vi "Binding Machine.vi"() -> ()   [LabVIEW 2014]
uses:
  Master/Master.lvclass
  Programming Logic/Programing Logic.lvclass
panel:
  out "Admin Enable":bool
  out "Drives Connection":cluster{"Drive 1":bool, "Drive 2":bool}
  in  "Delete All Record":bool
  in  "Select Record":u16(ring) items=["1", "2"]
  in  "Delete Record":bool
  out "NO.     User                   Date                 min   hr       Yields":T1(array[cluster])
  in  "Reconnect":bool
  in  "Tab Control 3":enum32{"Production", "Recipe", "Settings"}(tab)
  in  "Clear":bool
  in  "decrease":bool
  in  "Increase":bool
  out "User Yields":dbl
  in  "Zero Total Yields":bool
  out "Total Yields":dbl
  in  "Download":bool
  in  "Select Recipe":u16(ring) items=["1234567hjed", "tswri", "ad975t", "6yt"]
  in  "User 2":bool
  in  "User 1":bool
  in  "Start":bool
  in  "Stop":bool
  in  "Homing":bool
  in  "Jogging":bool
  out "Current Recipe":T2
  in  "Delete Selected Recipe":bool
  in  "Delete All Recipe":bool
  in  "Delete Recipe":u16(ring) items=["1234567hjed", "tswri", "ad975t", "6yt"]
  in  "Add Recipe":bool
  out "Index Name               Wind Leng.     Wind Spd.         Kink Cyc.        Bind Leng.        Unit":T3(array[cluster])
  in  "Set Production Page 2":bool
  in  "Set Jogging Speed":string
  in  "Display Recipe":bool
  in  "Set Auto Log off":bool
  in  "Auto Log off Time (min)":dbl
  in  "Set Admin Password":bool
  in  "Set Admin Password":T4
  out "Status":T5
  in  "Test":bool
  in  "Set Production Page":bool
  out "Time 3":dbl
  in  "Exit":bool
  out "error out":errorcluster
  in  "error in":errorcluster
  out "tab3":bool
  out "tab2":bool
  out "tab1":bool
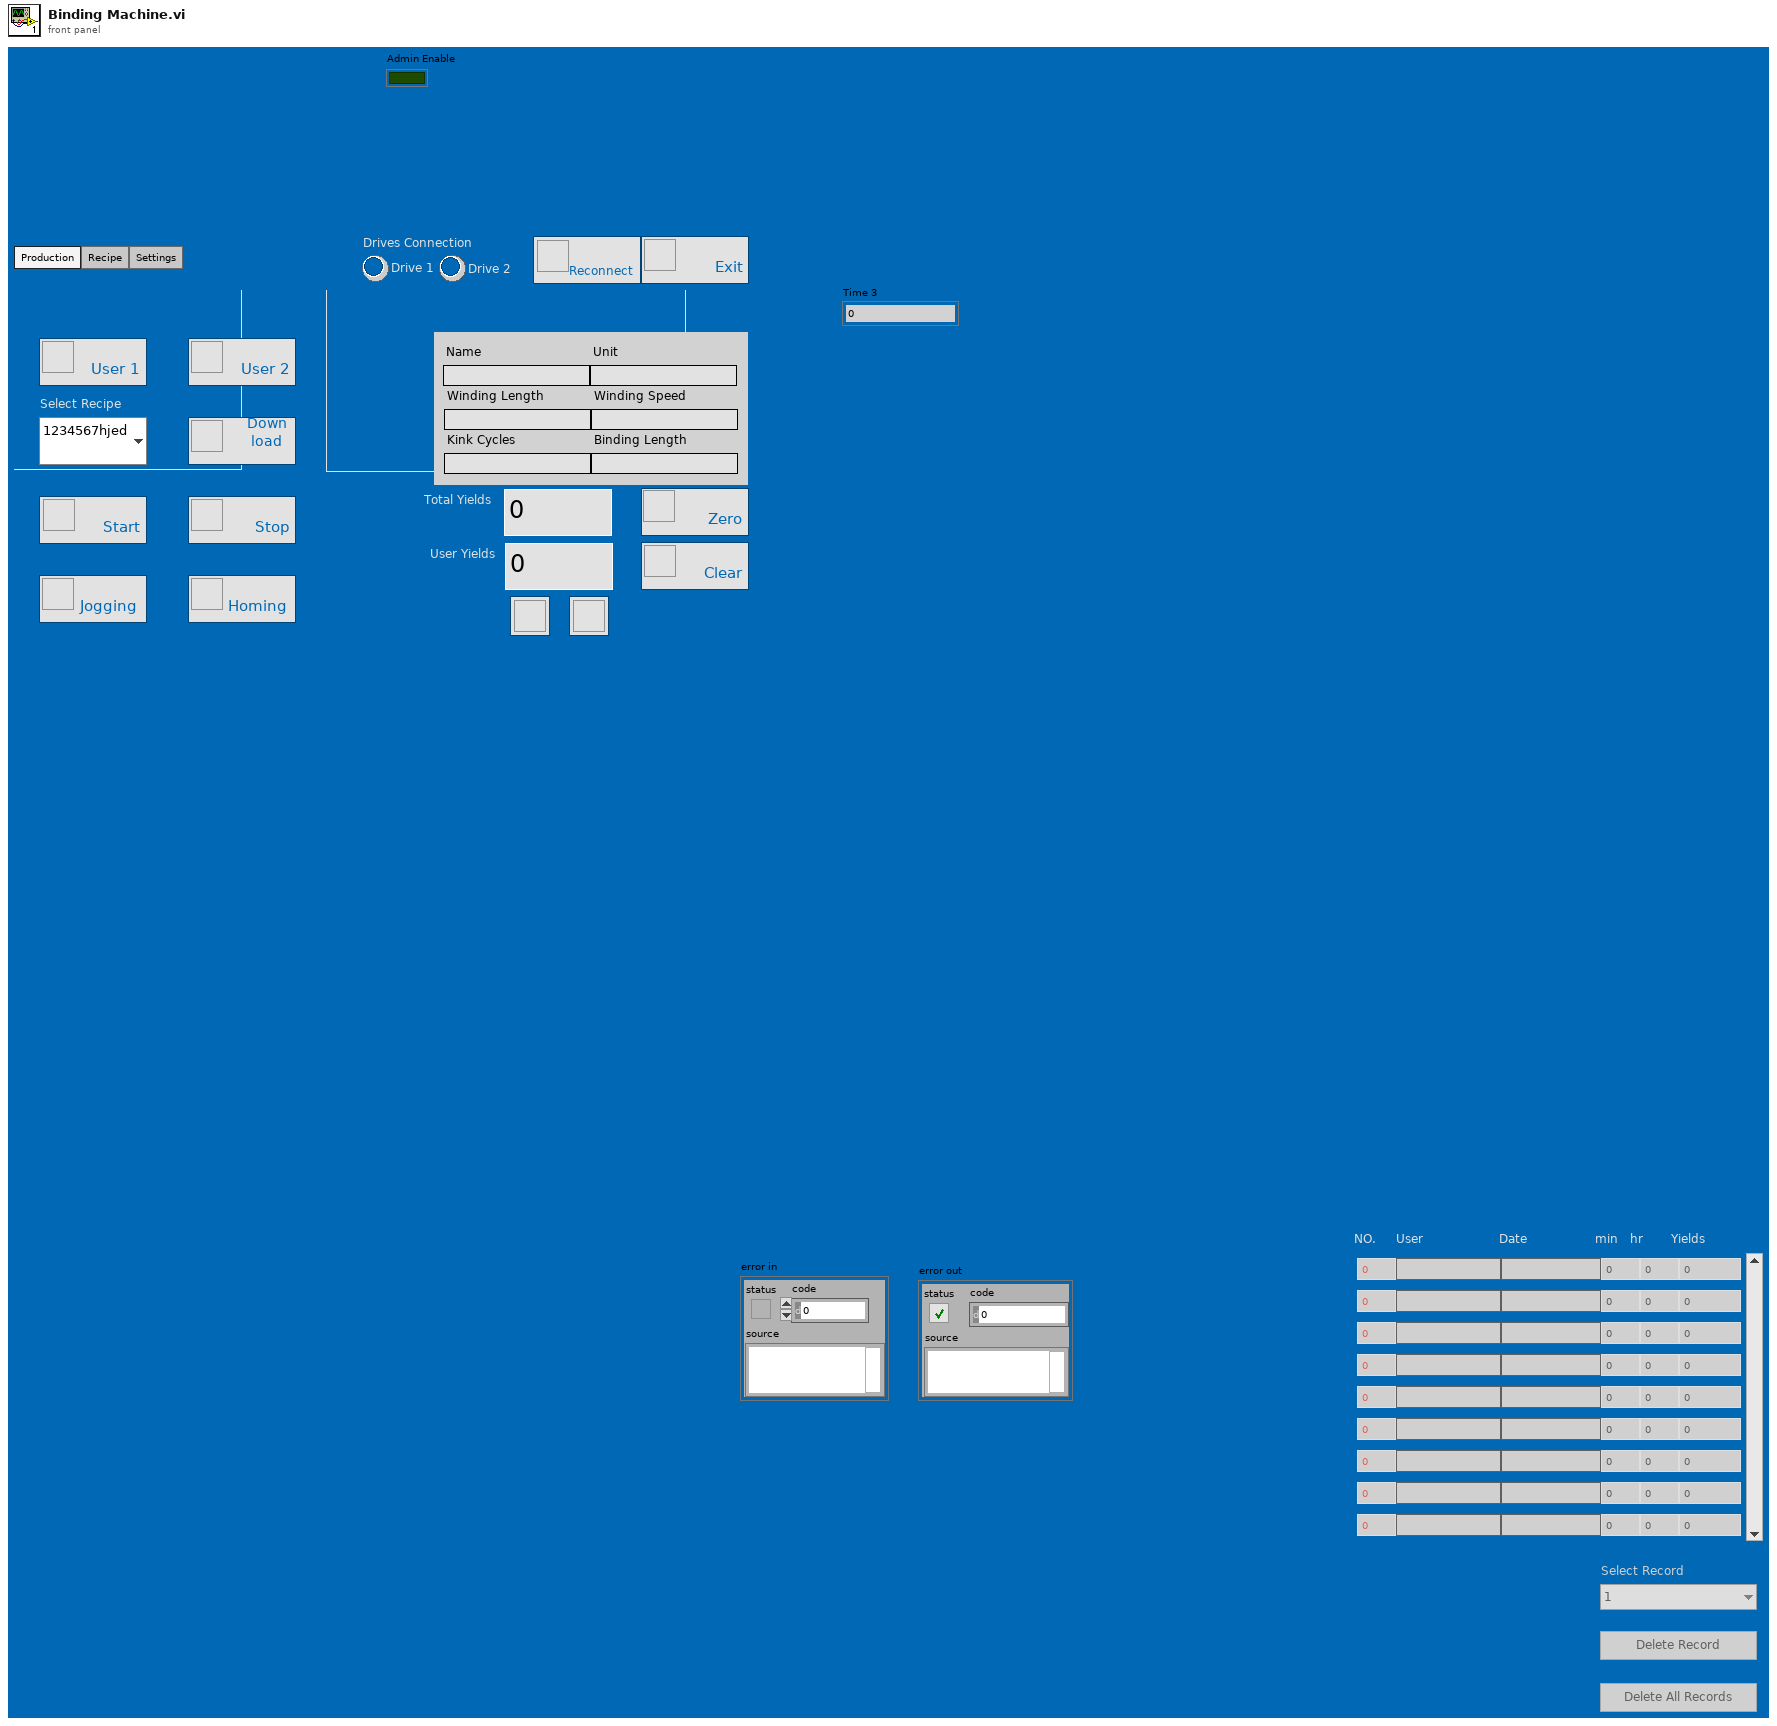
[diagram p1: front panel]
types:
  T1 = cluster{"index":i32, "User 2":string, "Date":string, "hour":i32, "min":i32, "Yields":dbl}[]
  T2 = cluster{"Name":string, "Winding Length":string, "Winding Speed":string, "Kink Cycles ":string, "Binding Length":string, "Unit":string}
  T3 = cluster{"NO.":dbl, "Name":string, "Winding Length":string, "Winding Speed":string, "Kink Cycles":string, "Binding Length":string, "Unit":string}[]
  T4 = cluster{"Old Admin Password":string, "New Admin Password":string, "Confirm  Password":string}
  T5 = cluster{"Winding":cluster{"Winding Unit":string, "Winding Speed":string, "Winding Length":string}, "Binding":cluster{"Binding Unit":string, "Kink Cycles":string, "Binding Length":string}, "Current Yields":dbl, "DataTime":cluster{"Date":string, "Time":string}, "Current User":string, "Minute":i32, "Hour":i32, "Drives Connection":cluster{"Drive 1":bool, "Drive 2":bool}}
  T6 = cluster{"Winding":cluster{"Winding Unit":string, "Winding Speed":string, "Winding Length":string}, "Binding":cluster{"Binding Unit":string, "Kink Cycles":string, "Binding Length":string}, "Yield Counts":dbl, "DataTime":cluster{"Date":string, "Time":string}, "User":string, "hour":i32, "minute":i32, "Drives Connection":cluster{"Drive 1":bool, "Drive 2":bool}}
  T7 = cluster{"Name":string, "Wind Length":string, "Wind Spd":string, "Kink Cyc":string, "Bind Length":string, "Unit":string}
  T8 = enum16{"record", "winding", "binding", "user", "recipe"}[]
  T9 = cluster{"Index":i32, "Name":string, "Wind Length":string, "Wind Spd":string, "Kink Cyc":string, "Bind Leng":string, "Unit":string}[]
  T10 = cluster{"index":i32, "User":string, "Date":string, "hour":i32, "minute":i32, "Yields":dbl}[]
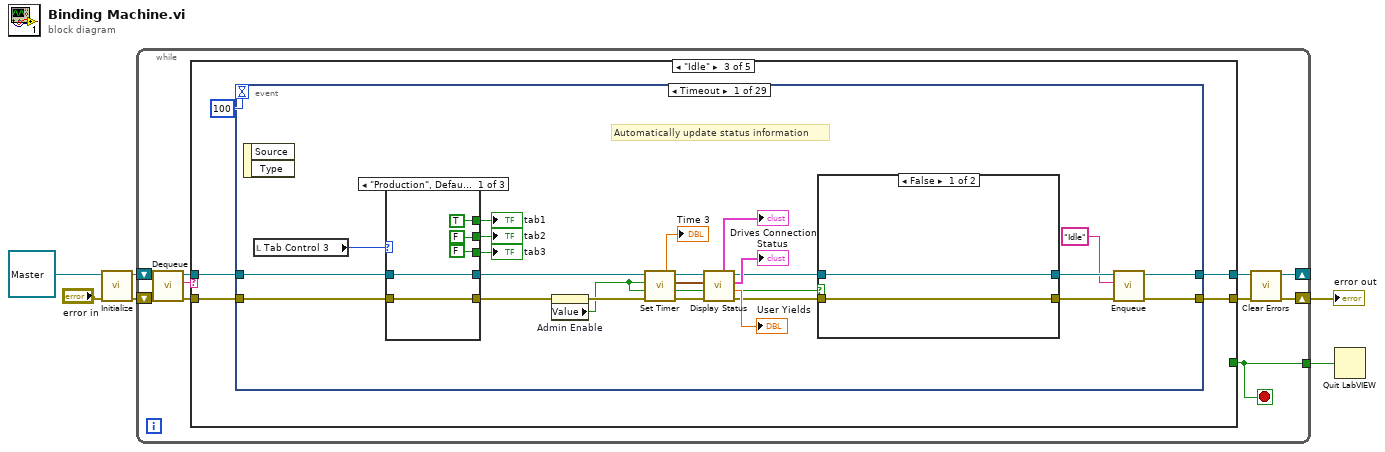
[diagram p0: block diagram]
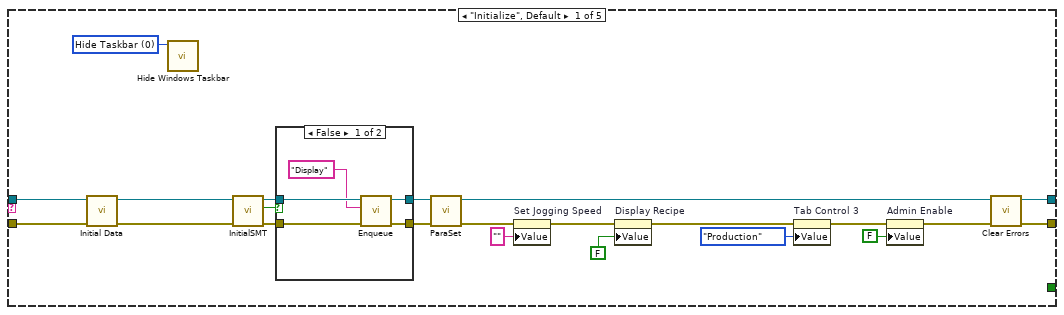
[diagram p2: hidden frame]
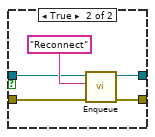
[diagram p3: hidden frame]
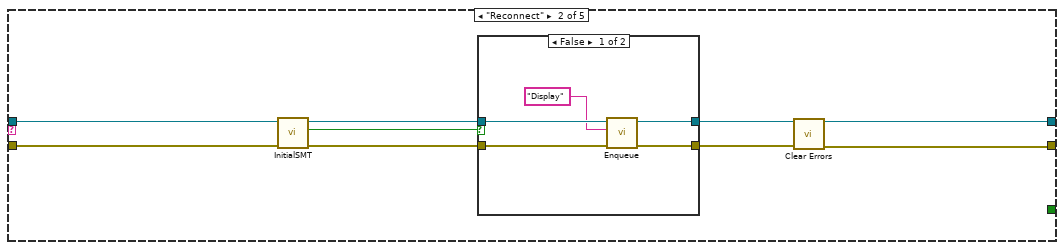
[diagram p4: hidden frame]
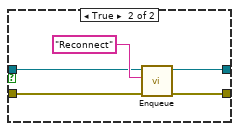
[diagram p5: hidden frame]
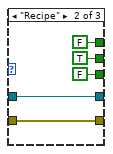
[diagram p6: hidden frame]
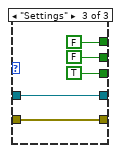
[diagram p7: hidden frame]
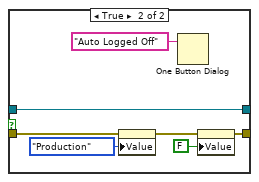
[diagram p8: hidden frame]
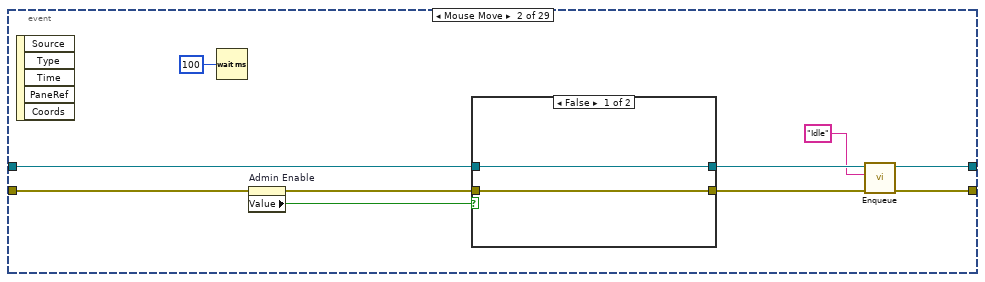
[diagram p9: hidden frame]
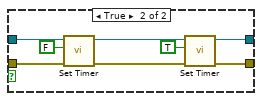
[diagram p10: hidden frame]
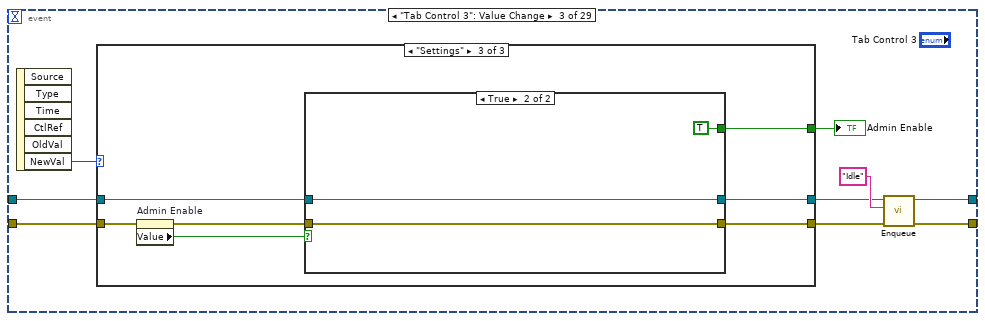
[diagram p11: hidden frame]
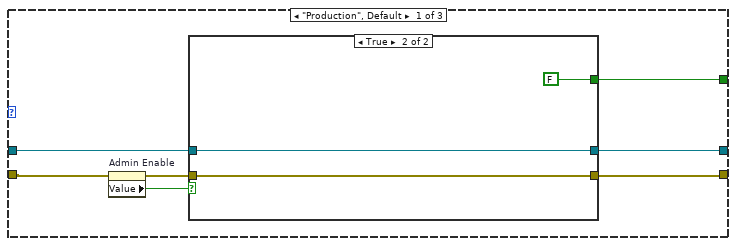
[diagram p12: hidden frame]
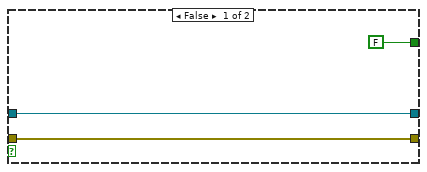
[diagram p13: hidden frame]
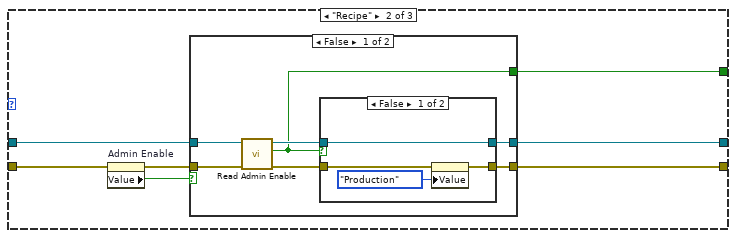
[diagram p14: hidden frame]
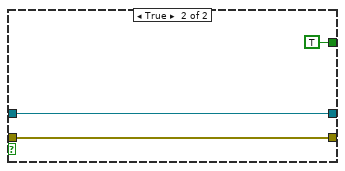
[diagram p16: hidden frame]
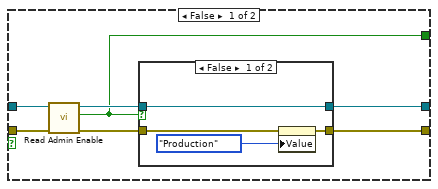
[diagram p17: hidden frame]
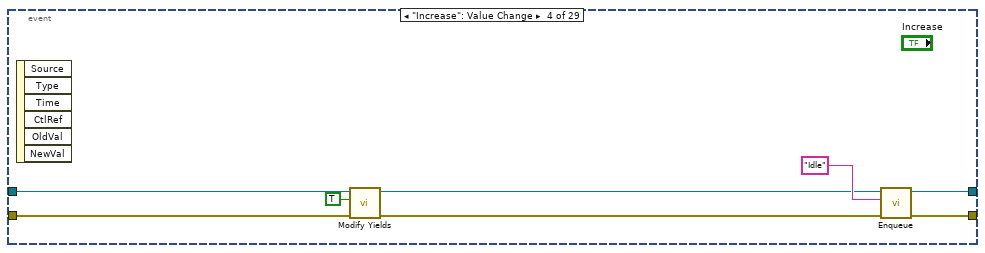
[diagram p19: hidden frame]
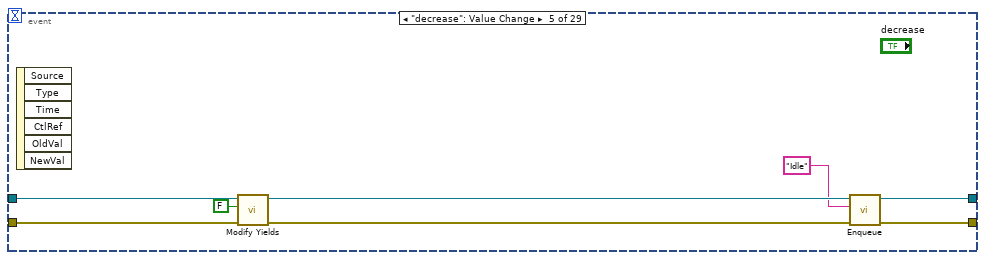
[diagram p20: hidden frame]
diagram:
  n1 = call-dynamic "Initialize.vi"("error in (no error)"="error in", "Master in"=refnum<class "Master.lvclass"> refnum ("Master.lvclass")) -> ("error out"=w4:errorcluster, "Master out"=w5:refnum<class "Master.lvclass">)  [unwired: 8 in]
  n2 = while {
    shift-right: [w11] -> _
    shift-left: w5 -> [w15]
    shift-right: [w7] -> w6
    shift-left: w4 -> [w14]
    tunnel: [w9] -> w1
    stop <- w9 stop-if-true
    n3 = call-dynamic "Dequeue.vi"("error in (no error)"=w14, "Master in"=w15) -> ("error out"=w10:errorcluster, "State"=w13:string, "Master out"=w12:refnum<class "Master.lvclass">)  [unwired: 7 in]
    n4 = case shown="\"Idle\"" w13 {
      tunnel: w12 -> [w36 w52 w69 w537 w568]
      tunnel: [w26 w50 w66 w532 w566] -> w11
      tunnel: w10 -> [w35 w51 w68 w536 w567]
      tunnel: [w16 w47 w67 w531 w565] -> w8
      tunnel: [_ _ _ _ TRUE] -> w9
      frame "Initialize", Default {
        w27 = u16 0 items=["Hide Taskbar", "Unhide Taskbar"] ("Operation")
        n5 = call-dynamic "Initial Data.vi"("error in (no error)"=w35, "Master in"=w36) -> ("error out"=w33:errorcluster, "Master out"=w34:refnum<class "Master.lvclass">)  [unwired: 8 in]
        n6 = call "Hide Windows Taskbar.vi"("Operation"=w27) -> ()  [unwired: 6 in, 1 out]
        n7 = call-dynamic "InitialSMT.vi"("error in (no error)"=w33, "Programing Logic in"=w34) -> ("error out"=w31:errorcluster, "Reconnect"=w30:bool, "Programing Logic out"=w32:refnum<class "Master.lvclass">)  [unwired: 7 in]
        n8 = case shown="False" w30 {
          tunnel: [w41 w45] -> w29
          tunnel: [w40 w44] -> w28
          tunnel: w32 -> [w39 w43]
          tunnel: w31 -> [w38 w42]
          frame False {
            n9 = call-dynamic "Enqueue.vi"("error in (no error)"=w38, "State"="Display", "Master in"=w39) -> ("error out"=w40:errorcluster, "Master out"=w41:refnum<class "Master.lvclass">)  [unwired: 7 in]
          }
          frame True {
            n10 = call-dynamic "Enqueue.vi"("error in (no error)"=w42, "State"="Reconnect", "Master in"=w43) -> ("error out"=w44:errorcluster, "Master out"=w45:refnum<class "Master.lvclass">)  [unwired: 7 in]
          }
        }
        n11 = call-dynamic "ParaSet.vi"("error in (no error)"=w28, "Programing Logic in"=w29) -> ("error out"=w22:errorcluster, "Programing Logic out"=w26:refnum<class "Master.lvclass">)  [unwired: 8 in]
        n12 = property on="Set Jogging Speed" class="Str"(error in=w22, "Value"="" ("Set Jogging Speed")) -> (error out=w21:errorcluster)  [unwired: 1 in, 1 out]
        n13 = property on="Display Recipe" class="Bool (strict)"(error in=w21, "Value"=FALSE ("Display Recipe")) -> (error out=w20:errorcluster)  [unwired: 1 in, 1 out]
        n14 = property on="Tab Control 3" class="TabCtl (strict)"(error in=w20, "Value"=enum32{"Production", "Recipe", "Settings"}."Production" ("Tab Control 3")) -> (error out=w24:errorcluster)  [unwired: 1 in, 1 out]
        n15 = property on="Admin Enable" class="Bool (strict)"(error in=w24, "Value"=FALSE ("Admin Enable")) -> (error out=w17:errorcluster)  [unwired: 1 in, 1 out]
        n16 = call <vilib>:"Clear Errors.vi"("error in (no error)"=w17) -> ("error out"=w16:errorcluster)  [unwired: 5 in, 1 out]
      }
      frame "Reconnect" {
        n17 = call-dynamic "InitialSMT.vi"("error in (no error)"=w51, "Programing Logic in"=w52) -> ("error out"=w53:errorcluster, "Reconnect"=w49:bool, "Programing Logic out"=w54:refnum<class "Master.lvclass">)  [unwired: 7 in]
        n18 = case shown="False" w49 {
          tunnel: w54 -> [w57 w63]
          tunnel: w53 -> [w56 w62]
          tunnel: [w59 w61] -> w50
          tunnel: [w58 w60] -> w48
          frame False {
            n19 = call-dynamic "Enqueue.vi"("error in (no error)"=w56, "State"="Display", "Master in"=w57) -> ("error out"=w58:errorcluster, "Master out"=w59:refnum<class "Master.lvclass">)  [unwired: 7 in]
          }
          frame True {
            n20 = call-dynamic "Enqueue.vi"("error in (no error)"=w62, "State"="Reconnect", "Master in"=w63) -> ("error out"=w60:errorcluster, "Master out"=w61:refnum<class "Master.lvclass">)  [unwired: 7 in]
          }
        }
        n21 = call <vilib>:"Clear Errors.vi"("error in (no error)"=w48) -> ("error out"=w47:errorcluster)  [unwired: 5 in, 1 out]
      }
      frame "Idle" {
        n22 = event shown="[0] Timeout" {
          selector: _ -> [_ _ _ _ _ _ _ _ _ _ _ _ _ _ _ _ _ _ _ _ _ _ _ _ _ _ _ _ _]
          dyn-events: _ -> [_ _ _ _ _ _ _ _ _ _ _ _ _ _ _ _ _ _ _ _ _ _ _ _ _ _ _ _ _]
          timeout: 100 -> [_ _ _ _ _ _ _ _ _ _ _ _ _ _ _ _ _ _ _ _ _ _ _ _ _ _ _ _ _]
          tunnel: w69 -> [w77 w127 w143 w214 w222 w224 w251 w262 w270 w284 w290 w298 w305 w312 w320 w322 w329 w344 w357 w377 w390 w407 w419 w435 w462 w498 w501 w509 w517]
          tunnel: w68 -> [w74 w124 w141 w213 w221 w223 w250 w261 w269 w275 w289 w294 w301 w308 w319 w321 w333 w343 w350 w370 w389 w406 w418 w434 w461 w497 w500 w507 w516]
          tunnel: [w82 w120 w146 w207 w217 w229 w252 w264 w272 w279 w285 w296 w303 w310 w316 w323 w331 w346 w354 w374 w391 w412 w427 w428 w467 w488 w504 w512 w521] -> w67
          tunnel: [w83 w121 w147 w208 w218 w230 w253 w265 w273 w280 w286 w297 w304 w311 w317 w324 w330 w347 w355 w375 w392 w411 w426 w429 w466 w489 w503 w511 w522] -> w66
          event Timeout {
            # "Automatically update status information"
            n23 = event-data() -> ()  [unwired: 1 in, 2 out]
            n24 = local read "Tab Control 3"() -> (w76:enum32{"Production", "Recipe", "Settings"})
            n25 = case shown="\"Production\", Default" w76 {
              tunnel: w77 -> [w99 w104 w109]
              tunnel: [w99 w104 w109] -> w75
              tunnel: [w98 w103 w108] -> w73
              tunnel: w74 -> [w98 w103 w108]
              tunnel: [TRUE FALSE FALSE] -> w72
              tunnel: [FALSE FALSE TRUE] -> w71
              tunnel: [FALSE TRUE FALSE] -> w70
              frame "Production", Default {
              }
              frame "Recipe" {
              }
              frame "Settings" {
              }
            }
            "tab1" <- w72
            "tab2" <- w70
            "tab3" <- w71
            n26 = property on="Admin Enable" class="Bool (strict)"(error in=w73) -> (error out=w86:errorcluster, "Value"=w85:bool)  [unwired: 1 in, 1 out]
            n27 = call-dynamic "Set Timer.vi"("error in (no error)"=w86, "User"=w85, "Admin"=w85, "Master in"=w75) -> ("error out"=w93:errorcluster, "Done"=w84:bool, "Cluster"=w92:cluster{"minute":i32, "hour":i32}, "Master out"=w94:refnum<class "Master.lvclass">, "Time"=→"Time 3":dbl)  [unwired: 2 in, 1 out]
            n28 = call-dynamic "Display Status.vi"("error in (no error)"=w93, "Status.Login Time"=w92, "Programing Logic in"=w94) -> ("error out"=w87:errorcluster, "commandValue"=→"User Yields":dbl, "Status"=→"Status":T6, "Programing Logic out"=w89:refnum<class "Master.lvclass">, "Drives Connection"=→"Drives Connection":cluster{"Drive 1":bool, "Drive 2":bool})  [unwired: 4 in]
            n29 = case shown="False" w84 {
              tunnel: [w110 w114] -> w80
              tunnel: [w111 w117] -> w81
              tunnel: w89 -> [w111 w117]
              tunnel: w87 -> [w110 w116]
              frame False {
              }
              frame True {
                n30 = property on="Tab Control 3" class="TabCtl (strict)"(error in=w116, "Value"=enum32{"Production", "Recipe", "Settings"}."Production" ("Tab Control 3")) -> (error out=w113:errorcluster)  [unwired: 1 in, 1 out]
                n31 = One Button Dialog(message="Auto Logged Off") -> ()  [unwired: 1 in, 1 out]
                n32 = property on="Admin Enable" class="Bool (strict)"(error in=w113, "Value"=FALSE ("Admin Enable")) -> (error out=w114:errorcluster)  [unwired: 1 in, 1 out]
              }
            }
            n33 = call-dynamic "Enqueue.vi"("error in (no error)"=w80, "State"="Idle", "Master in"=w81) -> ("error out"=w82:errorcluster, "Master out"=w83:refnum<class "Master.lvclass">)  [unwired: 7 in]
          }
          event Mouse Move {
            n34 = event-data() -> ()  [unwired: 1 in, 5 out]
            n35 = Wait (ms)(milliseconds to wait=u32 100) -> ()  [unwired: 1 out]
            n36 = property on="Admin Enable" class="Bool (strict)"(error in=w124) -> (error out=w123:errorcluster, "Value"=w125:bool)  [unwired: 1 in, 1 out]
            n37 = case shown="False" w125 {
              tunnel: w127 -> [w130 w138]
              tunnel: [w130 w136] -> w126
              tunnel: w123 -> [w129 w135]
              tunnel: [w129 w133] -> w122
              frame False {
              }
              frame True {
                n38 = call-dynamic "Set Timer.vi"("error in (no error)"=w135, "Admin"=FALSE, "Master in"=w138) -> ("error out"=w134:errorcluster, "Master out"=w137:refnum<class "Master.lvclass">)  [unwired: 3 in, 4 out]
                n39 = call-dynamic "Set Timer.vi"("error in (no error)"=w134, "Admin"=TRUE, "Master in"=w137) -> ("error out"=w133:errorcluster, "Master out"=w136:refnum<class "Master.lvclass">)  [unwired: 3 in, 4 out]
              }
            }
            n40 = call-dynamic "Enqueue.vi"("error in (no error)"=w122, "State"="Idle", "Master in"=w126) -> ("error out"=w120:errorcluster, "Master out"=w121:refnum<class "Master.lvclass">)  [unwired: 7 in]
          }
          event "Tab Control 3": Value Change {
            n41 = event-data() -> ("NewVal"=w144:enum32{"Production", "Recipe", "Settings"})  [unwired: 1 in, 5 out]
            n42 = case shown="\"Settings\"" w144 {
              tunnel: w143 -> [w152 w167 w189]
              tunnel: [w151 w166 w190] -> w142
              tunnel: w141 -> [w154 w164 w187]
              tunnel: [w149 w165 w185] -> w140
              tunnel: [w148 w161 w184] -> w139
              frame "Production", Default {
                n43 = property on="Admin Enable" class="Bool (strict)"(error in=w154) -> (error out=w150:errorcluster, "Value"=w153:bool)  [unwired: 1 in, 1 out]
                n44 = case shown="True" w153 {
                  tunnel: w152 -> [w157 w160]
                  tunnel: [w157 w160] -> w151
                  tunnel: [w156 w158] -> w149
                  tunnel: w150 -> [w156 w158]
                  tunnel: [FALSE ("Admin Enable") FALSE ("Admin Enable")] -> w148
                  frame False {
                  }
                  frame True {
                  }
                }
              }
              frame "Recipe" {
                n45 = property on="Admin Enable" class="Bool (strict)"(error in=w164) -> (error out=w163:errorcluster, "Value"=w162:bool)  [unwired: 1 in, 1 out]
                n46 = case shown="False" w162 {
                  tunnel: w167 -> [w174 w183]
                  tunnel: [w171 w183] -> w166
                  tunnel: [w169 w182] -> w165
                  tunnel: w163 -> [w173 w182]
                  tunnel: [w168 TRUE ("Admin Enable")] -> w161
                  frame False {
                    n47 = call-dynamic "Read Admin Enable.vi"("error in (no error)"=w173, "Master in"=w174) -> ("error out"=w170:errorcluster, "Admin Enable"=w168:bool, "Master out"=w172:refnum<class "Master.lvclass">)  [unwired: 4 in, 3 out]
                    n48 = case shown="False" w168 {
                      tunnel: [w178 w180] -> w171
                      tunnel: w172 -> [w178 w180]
                      tunnel: [w177 w179] -> w169
                      tunnel: w170 -> [w176 w179]
                      frame False {
                        n49 = property on="Tab Control 3" class="TabCtl (strict)"(error in=w176, "Value"=enum32{"Production", "Recipe", "Settings"}."Production" ("Tab Control 3")) -> (error out=w177:errorcluster)  [unwired: 1 in, 1 out]
                      }
                      frame True {
                      }
                    }
                  }
                  frame True {
                  }
                }
              }
              frame "Settings" {
                n50 = property on="Admin Enable" class="Bool (strict)"(error in=w187) -> (error out=w188:errorcluster, "Value"=w186:bool)  [unwired: 1 in, 1 out]
                n51 = case shown="True" w186 {
                  tunnel: w189 -> [w197 w206]
                  tunnel: [w194 w206] -> w190
                  tunnel: [w192 w205] -> w185
                  tunnel: w188 -> [w196 w205]
                  tunnel: [w191 TRUE ("Admin Enable")] -> w184
                  frame False {
                    n52 = call-dynamic "Read Admin Enable.vi"("error in (no error)"=w196, "Master in"=w197) -> ("error out"=w193:errorcluster, "Admin Enable"=w191:bool, "Master out"=w195:refnum<class "Master.lvclass">)  [unwired: 4 in, 3 out]
                    n53 = case shown="False" w191 {
                      tunnel: [w201 w203] -> w194
                      tunnel: w195 -> [w201 w203]
                      tunnel: [w200 w202] -> w192
                      tunnel: w193 -> [w199 w202]
                      frame False {
                        n54 = property on="Tab Control 3" class="TabCtl (strict)"(error in=w199, "Value"=enum32{"Production", "Recipe", "Settings"}."Production" ("Tab Control 3")) -> (error out=w200:errorcluster)  [unwired: 1 in, 1 out]
                      }
                      frame True {
                      }
                    }
                  }
                  frame True {
                  }
                }
              }
            }
            "Admin Enable" <- w139
            n55 = call-dynamic "Enqueue.vi"("error in (no error)"=w140, "State"="Idle", "Master in"=w142) -> ("error out"=w146:errorcluster, "Master out"=w147:refnum<class "Master.lvclass">)  [unwired: 7 in]
          }
          event "Increase": Value Change {
            n56 = event-data() -> ()  [unwired: 1 in, 6 out]
            n57 = call-dynamic "Modify Yields.vi"("error in (no error)"=w213, "Boolean"=TRUE, "Programing Logic in"=w214) -> ("error out"=w209:errorcluster, "Programing Logic out"=w210:refnum<class "Master.lvclass">)  [unwired: 7 in]
            n58 = call-dynamic "Enqueue.vi"("error in (no error)"=w209, "State"="Idle", "Master in"=w210) -> ("error out"=w207:errorcluster, "Master out"=w208:refnum<class "Master.lvclass">)  [unwired: 7 in]
          }
          event "decrease": Value Change {
            n59 = event-data() -> ()  [unwired: 1 in, 6 out]
            n60 = call-dynamic "Modify Yields.vi"("error in (no error)"=w221, "Boolean"=FALSE, "Programing Logic in"=w222) -> ("error out"=w219:errorcluster, "Programing Logic out"=w220:refnum<class "Master.lvclass">)  [unwired: 7 in]
            n61 = call-dynamic "Enqueue.vi"("error in (no error)"=w219, "State"="Idle", "Master in"=w220) -> ("error out"=w217:errorcluster, "Master out"=w218:refnum<class "Master.lvclass">)  [unwired: 7 in]
          }
          event "Zero Total Yields": Value Change {
            n62 = event-data() -> ()  [unwired: 1 in, 6 out]
            n63 = Two Button Dialog(message="Zero Total Yields?", 1:"No" ("F button name (\"Cancel\")"), 2:"Yes" ("T button name (\"OK\")")) -> (T button?=w228:bool)
            n64 = case shown="True" w228 {
              tunnel: [w234 w246] -> w230
              tunnel: [w233 w245] -> w229
              tunnel: w224 -> [w232 w237]
              tunnel: w223 -> [w231 w236]
              frame False {
                n65 = call-dynamic "Enqueue.vi"("error in (no error)"=w231, "State"="Idle", "Master in"=w232) -> ("error out"=w233:errorcluster, "Master out"=w234:refnum<class "Master.lvclass">)  [unwired: 7 in]
              }
              frame True {
                n66 = call-dynamic "Path.vi"("error in (no error)"=w236, "pathname"="production record", "Master in"=w237) -> ("error out"=w242:errorcluster, "Master out"=w243:refnum<class "Master.lvclass">)  [unwired: 7 in]
                n67 = call-dynamic "Zero Yields.vi"("error in (no error)"=w242, "Master in"=w243) -> ("error out"=w240:errorcluster, "Master out"=w241:refnum<class "Master.lvclass">)  [unwired: 8 in]
                n68 = call-dynamic "WriteFiles.vi"("error in (no error)"=w240, "Master in"=w241) -> ("error out"=w238:errorcluster, "Master out"=w239:refnum<class "Master.lvclass">)  [unwired: 8 in]
                n69 = call-dynamic "Enqueue.vi"("error in (no error)"=w238, "State"="Display", "Master in"=w239) -> ("error out"=w245:errorcluster, "Master out"=w246:refnum<class "Master.lvclass">)  [unwired: 7 in]
              }
            }
          }
          event "Clear": Value Change {
            n70 = event-data() -> ()  [unwired: 1 in, 6 out]
            n71 = call-dynamic "Zero.vi"("error in (no error)"=w250, "Programing Logic in"=w251) -> ("error out"=w248:errorcluster, "Programing Logic out"=w249:refnum<class "Master.lvclass">)  [unwired: 8 in]
            n72 = call-dynamic "Enqueue.vi"("error in (no error)"=w248, "Master in"=w249) -> ("error out"=w252:errorcluster, "Master out"=w253:refnum<class "Master.lvclass">)  [unwired: 8 in]
          }
          event "Set Auto Log off": Value Change {
            # "Set auto log off time by adminstrator only"
            n73 = event-data() -> ()  [unwired: 1 in, 6 out]
            n74 = call-dynamic "Set Auto Logoff.vi"("error in (no error)"=w261, "Timer.AutoLogoff"="Auto Log off Time (min)", "Master in"=w262) -> ("error out"=w259:errorcluster, "Master out"=w260:refnum<class "Master.lvclass">)  [unwired: 7 in]
            n75 = call-dynamic "Path.vi"("error in (no error)"=w259, "pathname"="login", "Master in"=w260) -> ("error out"=w257:errorcluster, "Master out"=w258:refnum<class "Master.lvclass">)  [unwired: 7 in]
            n76 = call-dynamic "WriteFiles.vi"("error in (no error)"=w257, "Master in"=w258) -> ("error out"=w255:errorcluster, "Master out"=w256:refnum<class "Master.lvclass">)  [unwired: 8 in]
            n77 = call-dynamic "Enqueue.vi"("error in (no error)"=w255, "State"="Idle", "Master in"=w256) -> ("error out"=w264:errorcluster, "Master out"=w265:refnum<class "Master.lvclass">)  [unwired: 7 in]
          }
          event "Add Recipe": Value Change {
            n78 = event-data() -> ()  [unwired: 1 in, 1 out]
            n79 = call-dynamic "Add Recipe.vi"("error in (no error)"=w269, "Master in"=w270) -> ("error out"=w267:errorcluster, "Master out"=w268:refnum<class "Master.lvclass">)  [unwired: 8 in]
            n80 = call-dynamic "Enqueue.vi"("error in (no error)"=w267, "State"="Display", "Master in"=w268) -> ("error out"=w272:errorcluster, "Master out"=w273:refnum<class "Master.lvclass">)  [unwired: 7 in]
          }
          event "Download": Value Change {
            n81 = event-data() -> ()  [unwired: 1 in, 1 out]
            n82 = call-dynamic "Download Recipe.vi"("index"="Select Recipe", "error in (no error)"=w275, "Master in"=w284) -> ("error out"=w281:errorcluster, "Parameter"=w282:T7, "Master out"=w283:refnum<class "Master.lvclass">)  [unwired: 6 in]
            n83 = call-dynamic "Download Recipe_galil.vi"("error in (no error)"=w281, "Parameter"=w282, "Programing Logic in"=w283) -> ("error out"=w276:errorcluster, "Programing Logic out"=w277:refnum<class "Master.lvclass">)  [unwired: 7 in]
            n84 = call-dynamic "Enqueue.vi"("error in (no error)"=w276, "State"="Display", "Master in"=w277) -> ("error out"=w279:errorcluster, "Master out"=w280:refnum<class "Master.lvclass">)  [unwired: 7 in]
          }
          event "Set Production Page 2": Value Change {
            n85 = event-data() -> ()  [unwired: 1 in, 1 out]
            n86 = call-dynamic "Display Recipe Enable.vi"("error in (no error)"=w289, "Display Recipe"="Display Recipe", "Master in"=w290) -> ("error out"=w287:errorcluster, "Master out"=w288:refnum<class "Master.lvclass">)  [unwired: 7 in]
            n87 = call-dynamic "Enqueue.vi"("error in (no error)"=w287, "State"="Display", "Master in"=w288) -> ("error out"=w285:errorcluster, "Master out"=w286:refnum<class "Master.lvclass">)  [unwired: 7 in]
          }
          event "Set Admin Password.Old Admin Password": Mouse Down {
            n88 = event-data() -> ()  [unwired: 1 in, 1 out]
            n89 = call "numberpad.vi"() -> ("String"=w293:string)  [unwired: 11 in]
            n90 = property on="Old Admin Password" class="Str"(error in=w294, "Value"=w293) -> (error out=w295:errorcluster)  [unwired: 1 in, 1 out]
            n91 = call-dynamic "Enqueue.vi"("error in (no error)"=w295, "State"="Idle", "Master in"=w298) -> ("error out"=w296:errorcluster, "Master out"=w297:refnum<class "Master.lvclass">)  [unwired: 7 in]
          }
          event "Set Admin Password.New Admin Password": Mouse Down {
            n92 = event-data() -> ()  [unwired: 1 in, 1 out]
            n93 = call "numberpad.vi"() -> ("String"=w300:string)  [unwired: 11 in]
            n94 = property on="New Admin Password" class="Str"(error in=w301, "Value"=w300) -> (error out=w302:errorcluster)  [unwired: 1 in, 1 out]
            n95 = call-dynamic "Enqueue.vi"("error in (no error)"=w302, "State"="Idle", "Master in"=w305) -> ("error out"=w303:errorcluster, "Master out"=w304:refnum<class "Master.lvclass">)  [unwired: 7 in]
          }
          event "Set Admin Password.Confirm  Password": Mouse Down {
            n96 = event-data() -> ()  [unwired: 1 in, 1 out]
            n97 = call "numberpad.vi"() -> ("String"=w307:string)  [unwired: 11 in]
            n98 = property on="Confirm  Password" class="Str"(error in=w308, "Value"=w307) -> (error out=w309:errorcluster)  [unwired: 1 in, 1 out]
            n99 = call-dynamic "Enqueue.vi"("error in (no error)"=w309, "State"="Idle", "Master in"=w312) -> ("error out"=w310:errorcluster, "Master out"=w311:refnum<class "Master.lvclass">)  [unwired: 7 in]
          }
          event "Test": Value Change {
            n100 = event-data() -> ()  [unwired: 1 in, 1 out]
            n101 = call-dynamic "Motor Test.vi"("error in (no error)"=w319, "Programing Logic in"=w320) -> ("error out"=w314:errorcluster, "Programing Logic out"=w315:refnum<class "Master.lvclass">)  [unwired: 8 in]
            n102 = call-dynamic "Enqueue.vi"("error in (no error)"=w314, "State"="Idle", "Master in"=w315) -> ("error out"=w316:errorcluster, "Master out"=w317:refnum<class "Master.lvclass">)  [unwired: 7 in]
          }
          event "Set Production Page": Value Change {
            n103 = event-data() -> ()  [unwired: 1 in, 1 out]
            n104 = call-dynamic "Set Jogging Spd.vi"("error in (no error)"=w321, "Set Jogging Speed"="Set Jogging Speed", "Programing Logic in"=w322) -> ("error out"=w325:errorcluster, "Programing Logic out"=w326:refnum<class "Master.lvclass">)  [unwired: 7 in]
            n105 = call-dynamic "Enqueue.vi"("error in (no error)"=w325, "State"="Display", "Master in"=w326) -> ("error out"=w323:errorcluster, "Master out"=w324:refnum<class "Master.lvclass">)  [unwired: 7 in]
          }
          event "Set Jogging Speed": Mouse Down {
            n106 = event-data() -> ()  [unwired: 1 in, 1 out]
            n107 = call "numberpad.vi"() -> ("String"=w334:string)  [unwired: 11 in]
            n108 = property on="Set Jogging Speed" class="Str"(error in=w333, "Value"=w334) -> (error out=w332:errorcluster)  [unwired: 1 in, 1 out]
            n109 = call-dynamic "Enqueue.vi"("error in (no error)"=w332, "State"="Idle", "Master in"=w329) -> ("error out"=w331:errorcluster, "Master out"=w330:refnum<class "Master.lvclass">)  [unwired: 7 in]
          }
          event "Delete Record": Value Change {
            n110 = event-data() -> ()  [unwired: 1 in, 1 out]
            n111 = call-dynamic "Path.vi"("error in (no error)"=w343, "pathname"="production record", "Master in"=w344) -> ("error out"=w339:errorcluster, "Master out"=w340:refnum<class "Master.lvclass">)  [unwired: 7 in]
            n112 = call-dynamic "Delete Record.vi"("index"="Select Record", "error in (no error)"=w339, "Master in"=w340) -> ("error out"=w337:errorcluster, "Master out"=w338:refnum<class "Master.lvclass">)  [unwired: 7 in]
            n113 = call-dynamic "WriteFiles.vi"("error in (no error)"=w337, "Master in"=w338) -> ("error out"=w341:errorcluster, "Master out"=w342:refnum<class "Master.lvclass">)  [unwired: 8 in]
            n114 = call-dynamic "Enqueue.vi"("error in (no error)"=w341, "State"="Display", "Master in"=w342) -> ("error out"=w346:errorcluster, "Master out"=w347:refnum<class "Master.lvclass">)  [unwired: 7 in]
          }
          event "User 1": Value Change {
            n115 = event-data() -> ()  [unwired: 1 in, 2 out]
            n116 = property on="User 1" class="Bool (strict)"(error in=w350) -> (error out=w351:errorcluster, "Value"=w349:bool)  [unwired: 1 in, 1 out]
            n117 = case shown="False" w349 {
              tunnel: w357 -> [w361 w367]
              tunnel: w351 -> [w359 w366]
              tunnel: [w360 w365] -> w353
              tunnel: [w361 w362] -> w352
              frame False {
                n118 = property on="User 1" class="Bool (strict)"(error in=w359, "Value"=TRUE ("User 1")) -> (error out=w360:errorcluster)  [unwired: 1 in, 1 out]
              }
              frame True {
                n119 = call-dynamic "Load User.vi"("User Name 2"="User 1", "error in (no error)"=w366, "Programing Logic in"=w367) -> ("error out"=w364:errorcluster, "Programing Logic out"=w362:refnum<class "Master.lvclass">)  [unwired: 7 in]
                n120 = property on="User 2" class="Bool (strict)"(error in=w364, "Value"=FALSE ("User 2")) -> (error out=w365:errorcluster)  [unwired: 1 in, 1 out]
              }
            }
            n121 = call-dynamic "Enqueue.vi"("error in (no error)"=w353, "State"="Idle", "Master in"=w352) -> ("error out"=w354:errorcluster, "Master out"=w355:refnum<class "Master.lvclass">)  [unwired: 7 in]
          }
          event "User 2": Value Change {
            n122 = event-data() -> ()  [unwired: 1 in, 2 out]
            n123 = property on="User 2" class="Bool (strict)"(error in=w370) -> (error out=w371:errorcluster, "Value"=w369:bool)  [unwired: 1 in, 1 out]
            n124 = case shown="False" w369 {
              tunnel: w377 -> [w381 w388]
              tunnel: w371 -> [w379 w387]
              tunnel: [w381 w385] -> w373
              tunnel: [w380 w384] -> w372
              frame False {
                n125 = property on="User 2" class="Bool (strict)"(error in=w379, "Value"=TRUE ("User 2")) -> (error out=w380:errorcluster)  [unwired: 1 in, 1 out]
              }
              frame True {
                n126 = call-dynamic "Load User.vi"("User Name 2"="User 2", "error in (no error)"=w387, "Programing Logic in"=w388) -> ("error out"=w383:errorcluster, "Programing Logic out"=w385:refnum<class "Master.lvclass">)  [unwired: 7 in]
                n127 = property on="User 1" class="Bool (strict)"(error in=w383, "Value"=FALSE ("User 2")) -> (error out=w384:errorcluster)  [unwired: 1 in, 1 out]
              }
            }
            n128 = call-dynamic "Enqueue.vi"("error in (no error)"=w372, "State"="Idle", "Master in"=w373) -> ("error out"=w374:errorcluster, "Master out"=w375:refnum<class "Master.lvclass">)  [unwired: 7 in]
          }
          event "Reconnect": Value Change {
            n129 = event-data() -> ()  [unwired: 1 in, 2 out]
            n130 = call-dynamic "InitialSMT.vi"("error in (no error)"=w389, "Programing Logic in"=w390) -> ("error out"=w394:errorcluster, "Reconnect"=w395:bool, "Programing Logic out"=w393:refnum<class "Master.lvclass">)  [unwired: 7 in]
            n131 = case shown="True" w395 {
              tunnel: w393 -> [w398 w404]
              tunnel: w394 -> [w397 w403]
              tunnel: [w400 w402] -> w392
              tunnel: [w399 w401] -> w391
              frame False {
                n132 = call-dynamic "Enqueue.vi"("error in (no error)"=w397, "State"="Display", "Master in"=w398) -> ("error out"=w399:errorcluster, "Master out"=w400:refnum<class "Master.lvclass">)  [unwired: 7 in]
              }
              frame True {
                n133 = call-dynamic "Enqueue.vi"("error in (no error)"=w403, "State"="Reconnect", "Master in"=w404) -> ("error out"=w401:errorcluster, "Master out"=w402:refnum<class "Master.lvclass">)  [unwired: 7 in]
              }
            }
          }
          event "Exit": Value Change {
            n134 = event-data() -> ()  [unwired: 1 in, 6 out]
            n135 = call "Emergency Stop.vi"("error in (no error)"=w406, "Programing Logic in"=w407) -> ("error out"=w408:errorcluster, "Programing Logic out"=w409:refnum<class "Master.lvclass">)  [unwired: 8 in]
            n136 = call-dynamic "Enqueue.vi"("error in (no error)"=w408, "State"="Exit", "Master in"=w409) -> ("error out"=w412:errorcluster, "Master out"=w411:refnum<class "Master.lvclass">)  [unwired: 7 in]
          }
          event "Set Admin Password": Value Change {
            n137 = event-data() -> ()  [unwired: 1 in, 1 out]
            n138 = call-dynamic "Set Admin Password.vi"("error in (no error)"=w418, "Set New Admin Password"="Set Admin Password", "Master in"=w419) -> ("error out"=w417:errorcluster, "Master out"=w420:refnum<class "Master.lvclass">)  [unwired: 7 in]
            n139 = call-dynamic "Path.vi"("error in (no error)"=w417, "pathname"="login" ("Recipes"), "Master in"=w420) -> ("error out"=w421:errorcluster, "Master out"=w422:refnum<class "Master.lvclass">)  [unwired: 7 in]
            n140 = call-dynamic "WriteFiles.vi"("error in (no error)"=w421, "Master in"=w422) -> ("error out"=w415:errorcluster, "Master out"=w423:refnum<class "Master.lvclass">)  [unwired: 8 in]
            n141 = property on="Set Admin Password" class="Clust (strict)"(error in=w415, "Value"=cluster{string, string, string} {"", "", ""}) -> (error out=w414:errorcluster)  [unwired: 1 in, 1 out]
            n142 = call-dynamic "Enqueue.vi"("error in (no error)"=w414, "State"="Idle", "Master in"=w423) -> ("error out"=w427:errorcluster, "Master out"=w426:refnum<class "Master.lvclass">)  [unwired: 7 in]
          }
          event "Delete All Recipe": Value Change {
            n143 = event-data() -> ()  [unwired: 1 in, 1 out]
            n144 = Two Button Dialog(message="Delete All Recipes?", 1:"No" ("F button name (\"Cancel\")"), 2:"Yes" ("T button name (\"OK\")")) -> (T button?=w433:bool)
            n145 = case shown="True" w433 {
              tunnel: w435 -> [w440 w451]
              tunnel: w434 -> [w439 w450]
              tunnel: [w440 w444] -> w431
              tunnel: [w439 w443] -> w430
              frame False {
              }
              frame True {
                n146 = local read "Index Name               Wind Leng.     Wind Spd.         Kink Cyc.        Bind Leng.        Unit"() -> (w448:T3)
                n147 = Array Size(array=w448) -> (size(s)=w449:i32)
                n148 = for {
                  N: w449 -> [_]
                  shift-right: [w456] -> w447
                  shift-left: w451 -> [w454]
                  shift-right: [w455] -> w446
                  shift-left: w450 -> [w453]
                  n149 = call-dynamic "Delete Recipe.vi"("error in (no error)"=w453, "index"=0, "Master in"=w454) -> ("error out"=w455:errorcluster, "Master out"=w456:refnum<class "Master.lvclass">)  [unwired: 7 in]
                }
                n150 = call-dynamic "Path.vi"("error in (no error)"=w446, "pathname"="Recipes", "Master in"=w447) -> ("error out"=w441:errorcluster, "Master out"=w442:refnum<class "Master.lvclass">)  [unwired: 7 in]
                n151 = call-dynamic "WriteFiles.vi"("error in (no error)"=w441, "Master in"=w442) -> ("error out"=w443:errorcluster, "Master out"=w444:refnum<class "Master.lvclass">)  [unwired: 8 in]
              }
            }
            n152 = call-dynamic "Enqueue.vi"("error in (no error)"=w430, "State"="Display", "Master in"=w431) -> ("error out"=w428:errorcluster, "Master out"=w429:refnum<class "Master.lvclass">)  [unwired: 7 in]
          }
          event "Delete All Record": Value Change {
            n153 = event-data() -> ()  [unwired: 1 in, 1 out]
            n154 = Two Button Dialog(message="Delete All Records?", 1:"No" ("F button name (\"Cancel\")"), 2:"Yes" ("T button name (\"OK\")")) -> (T button?=w457:bool)
            n155 = case shown="True" w457 {
              tunnel: [w468 w474] -> w464
              tunnel: [w469 w479] -> w463
              tunnel: w462 -> [w468 w478]
              tunnel: w461 -> [w469 w476]
              frame False {
              }
              frame True {
                n156 = local read "NO.     User                   Date                 min   hr       Yields"() -> (w470:T1)
                n157 = Array Size(array=w470) -> (size(s)=w471:i32)
                n158 = for {
                  N: w471 -> [_]
                  shift-right: [w484] -> w477
                  shift-left: w478 -> [w485]
                  shift-right: [w482] -> w475
                  shift-left: w476 -> [w483]
                  n159 = call-dynamic "Delete Record.vi"("index"=0, "error in (no error)"=w483, "Master in"=w485) -> ("error out"=w482:errorcluster, "Master out"=w484:refnum<class "Master.lvclass">)  [unwired: 7 in]
                }
                n160 = call-dynamic "Path.vi"("error in (no error)"=w475, "pathname"="production record", "Master in"=w477) -> ("error out"=w472:errorcluster, "Master out"=w473:refnum<class "Master.lvclass">)  [unwired: 7 in]
                n161 = call-dynamic "WriteFiles.vi"("error in (no error)"=w472, "Master in"=w473) -> ("error out"=w479:errorcluster, "Master out"=w474:refnum<class "Master.lvclass">)  [unwired: 8 in]
              }
            }
            n162 = call-dynamic "Enqueue.vi"("error in (no error)"=w463, "State"="Display", "Master in"=w464) -> ("error out"=w467:errorcluster, "Master out"=w466:refnum<class "Master.lvclass">)  [unwired: 7 in]
          }
          event "Delete Selected Recipe": Value Change {
            n163 = event-data() -> ()  [unwired: 1 in, 1 out]
            n164 = call-dynamic "Delete Recipe.vi"("error in (no error)"=w497, "index"="Delete Recipe", "Master in"=w498) -> ("error out"=w494:errorcluster, "Master out"=w495:refnum<class "Master.lvclass">)  [unwired: 7 in]
            n165 = call-dynamic "Path.vi"("error in (no error)"=w494, "pathname"="Recipes", "Master in"=w495) -> ("error out"=w492:errorcluster, "Master out"=w493:refnum<class "Master.lvclass">)  [unwired: 7 in]
            n166 = call-dynamic "WriteFiles.vi"("error in (no error)"=w492, "Master in"=w493) -> ("error out"=w490:errorcluster, "Master out"=w491:refnum<class "Master.lvclass">)  [unwired: 8 in]
            n167 = call-dynamic "Enqueue.vi"("error in (no error)"=w490, "State"="Display", "Master in"=w491) -> ("error out"=w488:errorcluster, "Master out"=w489:refnum<class "Master.lvclass">)  [unwired: 7 in]
          }
          event "Stop": Value Change {
            n168 = event-data() -> ()  [unwired: 1 in, 6 out]
            n169 = call "Emergency Stop.vi"("error in (no error)"=w500, "Programing Logic in"=w501) -> ("error out"=w499:errorcluster, "Programing Logic out"=w502:refnum<class "Master.lvclass">)  [unwired: 8 in]
            n170 = call-dynamic "Enqueue.vi"("error in (no error)"=w499, "State"="Idle", "Master in"=w502) -> ("error out"=w504:errorcluster, "Master out"=w503:refnum<class "Master.lvclass">)  [unwired: 7 in]
          }
          event "Start": Value Change {
            n171 = event-data() -> ()  [unwired: 1 in, 6 out]
            n172 = call-dynamic "Start.vi"("error in (no error)"=w507, "Jogging"="Jogging", "Programing Logic in"=w509) -> ("error out"=w508:errorcluster, "Programing Logic out"=w510:refnum<class "Master.lvclass">)  [unwired: 7 in]
            n173 = call-dynamic "Enqueue.vi"("Data"=w508, "State"="Idle", "Master in"=w510) -> ("error out"=w512:errorcluster, "Master out"=w511:refnum<class "Master.lvclass">)  [unwired: 7 in]
          }
          event "Homing": Value Change {
            n174 = event-data() -> ()  [unwired: 1 in, 6 out]
            n175 = call-dynamic "StopSMT1.vi"("error in (no error)"=w516, "Programing Logic in"=w517) -> ("error out"=w518:errorcluster, "Programing Logic out"=w519:refnum<class "Master.lvclass">)  [unwired: 8 in]
            n176 = call-dynamic "Reset.vi"("error in (no error)"=w518, "Programing Logic in"=w519) -> ("error out"=w514:errorcluster, "Programing Logic out"=w515:refnum<class "Master.lvclass">)  [unwired: 8 in]
            n177 = call-dynamic "Enqueue.vi"("error in (no error)"=w514, "State"="Idle", "Master in"=w515) -> ("error out"=w521:errorcluster, "Master out"=w522:refnum<class "Master.lvclass">)  [unwired: 7 in]
          }
        }
      }
      frame "Display" {
        w528 = T8 [enum."record", enum."winding", enum."binding", enum."user", enum."recipe"] items=["record", "winding", "binding", "user", "recipe"]
        # "To update information on display when changes are made"
        n178 = local read "Select Recipe"() -> (w524:u16)
        n179 = call-dynamic "Display Information.vi"("error in (no error)"=w536, "Select Recipe"=w524, "Master in"=w537) -> ("error out"=w530:errorcluster, "Total Yields"=→"Total Yields":dbl, "Recipe"=→"Index Name               Wind Leng.     Wind Spd.         Kink Cyc.        Bind Leng.        Unit":T9, "Master out"=w527:refnum<class "Master.lvclass">, "Parameter"=→"Current Recipe":T7, "Production Record"=→"NO.     User                   Date                 min   hr       Yields":T10)  [unwired: 3 in]
        n180 = for {
          shift-right: [w541] -> w529
          shift-left: w530 -> [w542]
          tunnel: w528 -> [w540] mode=indexing
          shift-right: [w538] -> w526
          shift-left: w527 -> [w539]
          n181 = case shown="\"record\", Default" w540 {
            tunnel: w542 -> [w548 w562]
            tunnel: [w546 w558] -> w541
            tunnel: w539 -> [w544 w563]
            tunnel: [w543 w561] -> w538
            frame "record", Default {
              n182 = local read "NO.     User                   Date                 min   hr       Yields"() -> (w549:T1)
              n183 = Array Size(array=w549) -> (size(s)=w550:i32)
              n184 = for {
                N: w550 -> [_]
                tunnel: [w555] -> w545 mode=concatenating
                shift-right: [w552] -> w547
                shift-left: w548 -> [w552]
                shift-right: [w551] -> w543
                shift-left: w544 -> [w551]
                i -> [w556]
                n185 = Increment(x=w556) -> (x+1=w554:i32)
                n186 = Number To Decimal String(number=w554) -> (decimal integer string=w553:string)  [unwired: 1 in]
                n187 = Build Array(w553) -> (w555:string[])
              }
              n188 = property on="Select Record" class="Ring (strict)"(error in=w547, "Strings []"=w545) -> (error out=w546:errorcluster)  [unwired: 1 in, 1 out]
            }
            frame "recipe" {
              n189 = call-dynamic "Auto Ring_recipe.vi"("error in (no error)"=w562, "Master in"=w563) -> ("error out"=w560:errorcluster, "Master out"=w561:refnum<class "Master.lvclass">, "Array"=w557:string[])  [unwired: 6 in, 1 out]
              n190 = property on="Select Recipe" class="Ring (strict)"(error in=w560, "Strings []"=w557) -> (error out=w559:errorcluster)  [unwired: 1 in, 1 out]
              n191 = property on="Delete Recipe" class="Ring (strict)"(error in=w559, "Strings []"=w557) -> (error out=w558:errorcluster)  [unwired: 1 in, 1 out]
            }
          }
        }
        n192 = call-dynamic "Enqueue.vi"("error in (no error)"=w529, "State"="Idle", "Master in"=w526) -> ("error out"=w531:errorcluster, "Master out"=w532:refnum<class "Master.lvclass">)  [unwired: 7 in]
      }
      frame "Exit" {
        w564 = u16 1 items=["Hide Taskbar", "Unhide Taskbar"] ("Operation")
        n193 = call "Hide Windows Taskbar.vi"("Operation"=w564) -> ()  [unwired: 6 in, 1 out]
        n194 = call-dynamic "Release.vi"("error in (no error)"=w567, "Master in"=w568) -> ("error out"=w565:errorcluster, "Master out"=w566:refnum<class "Master.lvclass">)  [unwired: 8 in]
      }
    }
    n195 = call <vilib>:"Clear Errors.vi"("error in (no error)"=w8) -> ("error out"=w7:errorcluster)  [unwired: 5 in, 1 out]
  }
  "error out" <- w6
  n196 = Quit LabVIEW(quit? (T)=w1) -> ()
